vi "Theta 2.vi"(5 "XYZ_60":dbl[](array[numeric])=[0.0, 0.0, 0.0], 7 "XYZ_560":dbl[](array[numeric])=[0.0, 0.0, 0.0], 9 "XYZ_0":dbl[](array[numeric])=[0.0, 0.0, 0.0], 10 "theta_0":dbl, 11 "6R Type 3 Serial Arm Class in":refnum<class "NI_Robotics_6R Type 3 Serial Arm Class.lvclass">) -> (0 "AB":dbl[](array[numeric]), 1 "valid?":bool, 2 "theta_0 array":dbl[](array[numeric]), 3 "6R Type 3 Serial Arm Class out":refnum<class "NI_Robotics_6R Type 3 Serial Arm Class.lvclass">)   [LabVIEW 2017, in "NI_Robotics_6R Type 3 Serial Arm Class.lvclass"]
uses:
  <vilib>/robotics/Kinematics/Analytical/6R/Type 3/NI_Robotics_6R Type 3 Serial Arm Class.lvclass
  c:/Program Files (x86)/National Instruments/LabVIEW 2017/vi.lib/robotics/Kinematics/Analytical/Generic/NI_Robotics_Analytical Serial Arm Class.lvclass
  <vilib>/robotics/Kinematics/Analytical/Generic/NI_Robotics_Analytical Serial Arm Class.lvclass
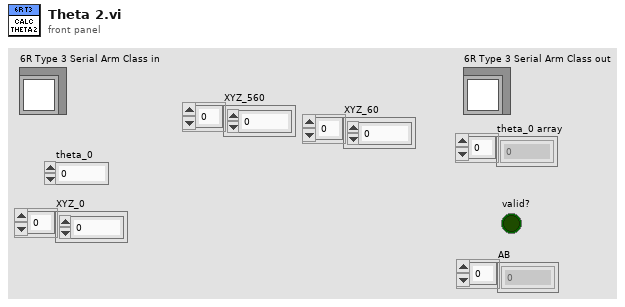
[diagram p1: front panel]
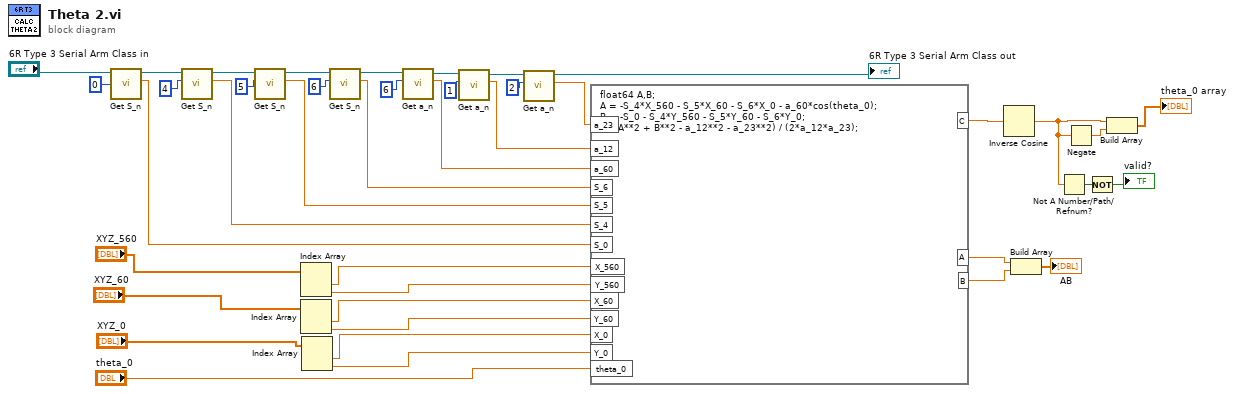
[diagram p0: block diagram]
diagram:
  n1 = call <vilib>:"Get S_n.vi"("n"=0, "Analytical Serial Arm Class in"="6R Type 3 Serial Arm Class in") -> ("S_n"=w24:dbl, "Analytical Serial Arm Class out"=w35:refnum<class "NI_Robotics_6R Type 3 Serial Arm Class.lvclass">)  [unwired: 8 in]
  n2 = call <vilib>:"Get S_n.vi"("n"=4, "Analytical Serial Arm Class in"=w35) -> ("S_n"=w22:dbl, "Analytical Serial Arm Class out"=w34:refnum<class "NI_Robotics_6R Type 3 Serial Arm Class.lvclass">)  [unwired: 8 in]
  n3 = call <vilib>:"Get S_n.vi"("n"=5, "Analytical Serial Arm Class in"=w34) -> ("S_n"=w21:dbl, "Analytical Serial Arm Class out"=w33:refnum<class "NI_Robotics_6R Type 3 Serial Arm Class.lvclass">)  [unwired: 8 in]
  n4 = Index Array(array="XYZ_560") -> (element #1=w18:dbl, element #2=w17:dbl)  [unwired: 2 in]
  n5 = Index Array(array="XYZ_60") -> (element #1=w26:dbl, element #2=w25:dbl)  [unwired: 2 in]
  n6 = Index Array(array="XYZ_0") -> (element #1=w29:dbl, element #2=w28:dbl)  [unwired: 2 in]
  n7 = call <vilib>:"Get S_n.vi"("n"=6, "Analytical Serial Arm Class in"=w33) -> ("S_n"=w20:dbl, "Analytical Serial Arm Class out"=w32:refnum<class "NI_Robotics_6R Type 3 Serial Arm Class.lvclass">)  [unwired: 8 in]
  n8 = call <vilib>:"Get a_n.vi"("n"=6, "Analytical Serial Arm Class in"=w32) -> ("a_n"=w19:dbl, "Analytical Serial Arm Class out"=w16:refnum<class "NI_Robotics_6R Type 3 Serial Arm Class.lvclass">)  [unwired: 8 in]
  n9 = call <vilib>:"Get a_n.vi"("n"=1, "Analytical Serial Arm Class in"=w16) -> ("a_n"=w12:dbl, "Analytical Serial Arm Class out"=w15:refnum<class "NI_Robotics_6R Type 3 Serial Arm Class.lvclass">)  [unwired: 8 in]
  n10 = call <vilib>:"Get a_n.vi"("n"=2, "Analytical Serial Arm Class in"=w15) -> ("a_n"=w11:dbl, "Analytical Serial Arm Class out"=→"6R Type 3 Serial Arm Class out":refnum<class "NI_Robotics_6R Type 3 Serial Arm Class.lvclass">)  [unwired: 8 in]
  n11 = formula code="float64 A,B;\nA = -S_4*X_560 - S_5*X_60 - S_6*X_0 - a_60*cos(theta_0);\nB = -S_0 - S_4*Y_560 - S_5*Y_60 - S_6*Y_0;\nC=(A**2 + B**2 - a_12**2 - a_23**2) / (2*a_12*a_23);"("a_60"=w19, "S_6"=w20, "S_5"=w21, "S_4"=w22, "S_0"=w24, "X_560"=w18, "Y_560"=w17, "X_60"=w26, "Y_60"=w25, "X_0"=w29, "Y_0"=w28, "theta_0"="theta_0", "a_12"=w12, "a_23"=w11) -> ("C"=w9:dbl, "A"=w3:dbl, "B"=w2:dbl)
  n12 = Inverse Cosine(1:w9) -> (0:w5:dbl)
  n13 = Build Array(w3, w2) -> (→"AB":dbl[])
  n14 = Not A Number/Path/Refnum?(number/path/refnum=w5) -> (NaN/Path/Refnum?=w7:bool)
  n15 = Negate(x=w5) -> (-x=w6:dbl)
  n16 = Not(x=w7) -> (.not. x?=→"valid?":bool)
  n17 = Build Array(w5, w6) -> (→"theta_0 array":dbl[])
